vi "Calling Class Methods.vi"() -> ()   [LabVIEW 2020]
uses:
  6d5f1638-640c-4e20-b011-0cee3ae60b95.vi
  688a6956-cd2d-4b8a-a8be-e172edc5432f.vi
  2e819b81-fe13-4050-befc-599fc726c07c.vi
  G-Embedded-Python-Interpreter-Toolkit/Null Py Object Refnum.vi
  6d5f1638-640c-4e20-b011-0cee3ae60b95.vi/96ddca92-7bbf-40e2-a1a5-d32f291eb6af.vi
  688a6956-cd2d-4b8a-a8be-e172edc5432f.vi/6c7a13f1-33d3-431d-8188-904cac5422b3.vi
  G-Embedded-Python-Interpreter-Toolkit/Python Object Reference to Pointer Sized Ref.vi
  2e819b81-fe13-4050-befc-599fc726c07c.vi/6c7a13f1-33d3-431d-8188-904cac5422b3.vi
  G-Embedded-Python-Interpreter-Toolkit/Pointer Sized Ref to Python Object Reference.vi
  G-Embedded-Python-Interpreter-Toolkit/Generate Function Call Argument Info.vi
  G-Embedded-Python-Interpreter-Toolkit/Bad Type Error.vi
  G-Embedded-Python-Interpreter-Toolkit/Generate Function Call Argument Info.vi/5ba79b4d-2978-48e4-80f3-d9d30d92ebfd.vi
  G-Embedded-Python-Interpreter-Toolkit/Merge Call Library Errors.vi
  <vilib>/Utility/Data Type/Get Type Information.vi
  <vilib>/Utility/error.llb/Error Cluster From Error Code.vi
  <vilib>/Utility/Data Type/Get Cluster Information.vi
  <vilib>/Utility/Data Type/Get Array Information.vi
  <vilib>/Comparison/Equal/Equal Functor/Equal Functor.lvclass
  G-Embedded-Python-Interpreter-Toolkit/G-Embedded-Python-Interpreter-Toolkit.lvlib
panel:
  in  "Decrement":bool
  in  "Increment":bool
  out "Counter Value":i32 format="%011d"
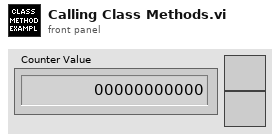
[diagram p1: front panel]
types:
  T1 = typedef "G-Embedded-Python-Interpreter-Toolkit.lvlib/Python Object Reference.ctl" = refnum<k1>
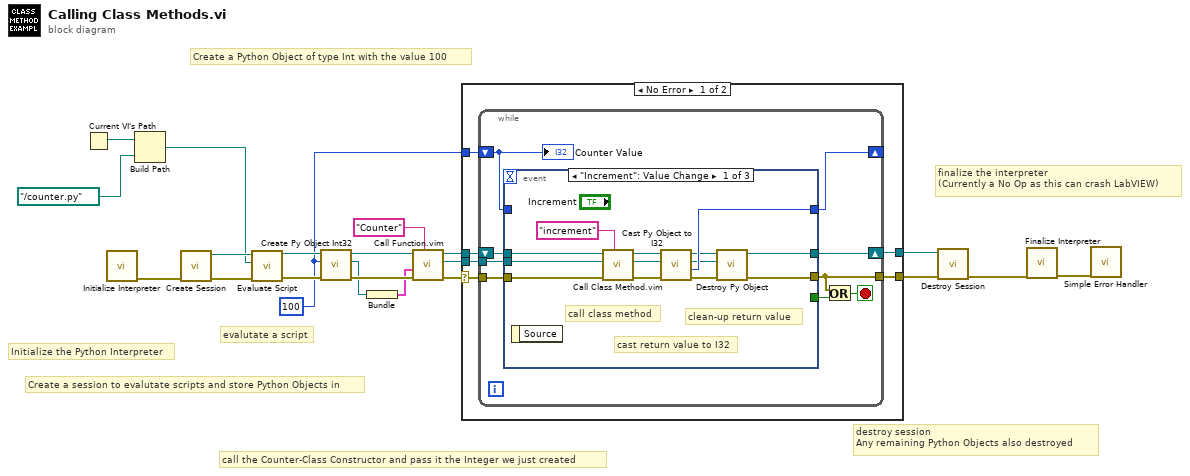
[diagram p0: block diagram]
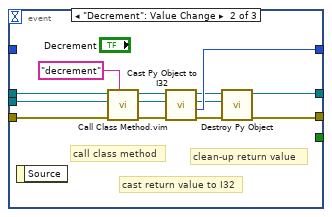
[diagram p2: hidden frame]
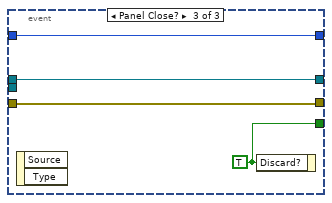
[diagram p3: hidden frame]
diagram:
  w10 = 100 ("Value")
  # "finalize the interpreter\n(Currently a No Op as this can crash LabVIEW)"
  # "destroy session \nAny remaining Python Objects also destroyed"
  # "Create a Python Object of type Int with the value 100"
  # "call the Counter-Class Constructor and pass it the Integer we just created"
  # "evalutate a script"
  # "Create a session to evalutate scripts and store Python Objects in"
  # "Initialize the Python Interpreter"
  n1 = Current VI's Path() -> (path=w18:path)
  n2 = call "Initialize Interpreter.vi"() -> ("error out"=w21:errorcluster)  [unwired: 10 in, 1 out]
  n3 = Build Path(base path=w18, name or relative path=path "../counter.py") -> (appended path=w16:path)
  n4 = call "Create Session.vi"("error in (no error)"=w21) -> ("error out"=w20:errorcluster, "Session Handle"=w19:refnum<data-value>)  [unwired: 9 in]
  n5 = call "Evaluate Script.vi"("error in (no error)"=w20, "Script File Path"=w16, "Session Handle in"=w19) -> ("error out"=w13:errorcluster, "Session Handle out"=w14:refnum<data-value>)  [unwired: 7 in]
  n6 = call "Create Py Object Int32.vi"("error in (no error)"=w13, "Value"=w10, "Session Handle in"=w14) -> ("error out"=w12:errorcluster, "Python Object Refnum"=w2:T1, "Session Handle out"=w11:refnum<data-value>)  [unwired: 6 in]
  n7 = Bundle("Python Object Refnum"=w2) -> (w1:cluster{"Python Object Refnum":T1})  [unwired: 1 in]
  n8 = call "Call Function.vim"("Function Name"="Counter", "error in (no error)"=w12, "Arguments in (Default - None)"=w1, "Data Value Reference in"=w11) -> ("error out"=w9:errorcluster, "Returned Python Object Refnum"=w7:T1, "Data Value Reference out"=w8:refnum<data-value>)  [unwired: 5 in]
  n9 = case shown="No Error" w9 {
    selector: w9 -> [w26 w68]
    tunnel: w10 -> [w27 _]
    tunnel: w8 -> [w25 w67]
    tunnel: w7 -> [w24 _]
    tunnel: [w23 w68] -> w6
    tunnel: [w22 w67] -> w5
    frame No Error {
      n10 = while {
        tunnel: w26 -> [w36]
        shift-right: [w31] -> w22
        shift-left: w25 -> [w35]
        tunnel: w24 -> [w34]
        shift-right: [w33] -> _
        shift-left: w27 -> [w30]
        tunnel: [w28] -> w23
        stop <- w32 stop-if-true
        n11 = event shown="[0] \"Increment\": Value Change" {
          selector: _ -> [_ _ _]
          dyn-events: _ -> [_ _ _]
          timeout: _ -> [_ _ _]
          tunnel: w36 -> [w49 w62 w66]
          tunnel: w35 -> [w48 w61 w65]
          tunnel: w34 -> [w47 w60 _]
          tunnel: [w42 w55 w64] -> w33
          tunnel: [w38 w51 w66] -> w28
          tunnel: [w37 w50 w65] -> w31
          tunnel: w30 -> [_ _ w64]
          tunnel: [_ _ w63] -> w29
          event "Increment": Value Change {
            # "clean-up return value"
            # "cast return value to I32"
            # "call class method"
            n12 = event-data() -> ()  [unwired: 1 in, 1 out]
            n13 = call "Call Class Method.vim"("Function Name"="increment", "error in (no error)"=w49, "Class Instance"=w47, "Data Value Reference in"=w48) -> ("error out"=w45:errorcluster, "Returned Python Object Refnum"=w43:T1, "Data Value Reference out"=w44:refnum<data-value>)  [unwired: 5 in]
            n14 = call "Cast Py Object to I32.vi"("error in (no error)"=w45, "Python Object Refnum in"=w43, "Session Handle in"=w44) -> ("error out"=w39:errorcluster, "Value"=w42:i32, "Python Object Refnum out"=w40:T1, "Session Handle out"=w41:refnum<data-value>)  [unwired: 5 in]
            n15 = call "Destroy Py Object.vi"("error in (no error)"=w39, "Python Object Refnum"=w40, "Session Handle in"=w41) -> ("error out"=w38:errorcluster, "Session Handle out"=w37:refnum<data-value>)  [unwired: 7 in]
          }
          event "Decrement": Value Change {
            # "clean-up return value"
            # "cast return value to I32"
            # "call class method"
            n16 = event-data() -> ()  [unwired: 1 in, 1 out]
            n17 = call "Call Class Method.vim"("Function Name"="decrement", "error in (no error)"=w62, "Class Instance"=w60, "Data Value Reference in"=w61) -> ("error out"=w58:errorcluster, "Returned Python Object Refnum"=w56:T1, "Data Value Reference out"=w57:refnum<data-value>)  [unwired: 5 in]
            n18 = call "Cast Py Object to I32.vi"("error in (no error)"=w58, "Python Object Refnum in"=w56, "Session Handle in"=w57) -> ("error out"=w52:errorcluster, "Value"=w55:i32, "Python Object Refnum out"=w53:T1, "Session Handle out"=w54:refnum<data-value>)  [unwired: 5 in]
            n19 = call "Destroy Py Object.vi"("error in (no error)"=w52, "Python Object Refnum"=w53, "Session Handle in"=w54) -> ("error out"=w51:errorcluster, "Session Handle out"=w50:refnum<data-value>)  [unwired: 7 in]
          }
          event Panel Close? {
            w63 = TRUE ("Discard?")
            n20 = event-data() -> ()  [unwired: 1 in, 2 out]
            n21 = event-data("Discard?"=w63) -> ()  [unwired: 1 in, 1 out]
          }
        }
        n22 = Or(x=w28, y=w29) -> (x .or. y?=w32:bool)
        "Counter Value" <- w30
      }
    }
    frame Error {
    }
  }
  n23 = call "Destroy Session.vi"("error in (no error)"=w6, "Session Handle"=w5) -> ("error out"=w4:errorcluster)  [unwired: 9 in]
  n24 = call "Finalize Interpreter.vi"("error in (no error)"=w4) -> ("error out"=w3:errorcluster)  [unwired: 10 in]
  n25 = call <vilib>:"Simple Error Handler.vi"("error in (no error)"=w3) -> ()  [unwired: 4 in, 5 out]
